vi "isReady.vi"(8 "error in (no error)":errorcluster, 11 "ExperimentControl in":refnum<class "ExperimentControl.lvclass">) -> (0 "error out":errorcluster, 2 "ready?":bool, 3 "ExperimentControl out":refnum<class "ExperimentControl.lvclass">)   [LabVIEW 2011, in "Views.lvlib" / "ExperimentControl.lvlib" / "ExperimentControl.lvclass"]
uses:
  ExperimentControl.lvclass
  ExperimentControl.lvclass/ExperimentControl.ctl
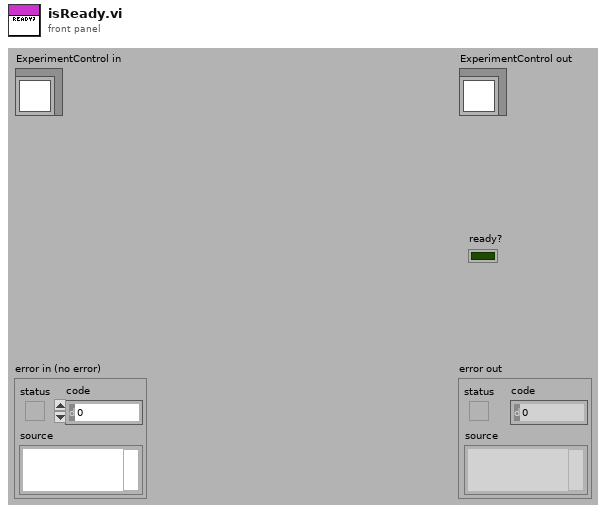
[diagram p1: front panel]
types:
  T1 = enum16{"Ready", "Compiling", "Configured", "Running", "Stopping", "Unresolved Error"}
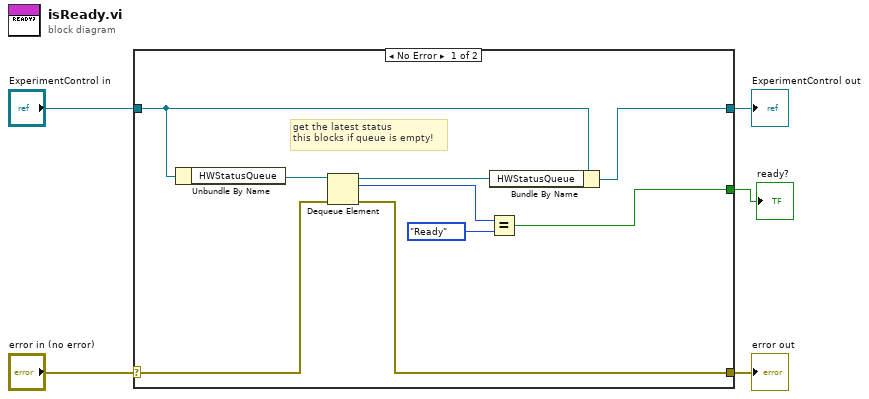
[diagram p0: block diagram]
diagram:
  n1 = case shown="No Error" "error in (no error)" {
    selector: "error in (no error)" -> [w13 w16]
    tunnel: [w12 w16] -> w4
    tunnel: [w7 w15] -> w2
    tunnel: "ExperimentControl in" -> [w8 w15]
    tunnel: [w9 _] -> w1
    frame No Error {
      # "get the latest status\nthis blocks if queue is empty!"
      n2 = Unbundle By Name(w8) -> ("HWStatusQueue"=w14:refnum<queue>)
      n3 = Dequeue Element(queue=w14, error in (no error)=w13) -> (queue out=w6:refnum<queue>, element=w11:T1, error out=w12:errorcluster)  [unwired: 1 in, 1 out]
      n4 = Equal?(x=w11, y=T1."Ready" ("element")) -> (x = y?=w9:bool)
      n5 = Bundle By Name(cluster=w8, "HWStatusQueue"=w6) -> (w7:refnum<class "ExperimentControl.lvclass">)
    }
    frame Error {
    }
  }
  "error out" <- w4
  "ExperimentControl out" <- w2
  "ready?" <- w1
